vi "Get Instruments.vi"(8 "error in (no error)":errorcluster, 11 "Test Class in":refnum<class "Test Class.lvclass">) -> (0 "error out":errorcluster, 3 "Instruments":refnum<class "Instrument.lvclass">[](array[class]))   [LabVIEW 2017, in "Test Class.lvclass"]
uses:
  Test Class.lvclass
  Classes/Instruments/Instrument/Class/Instrument.lvclass
  Classes/Application/Class/Application.lvclass
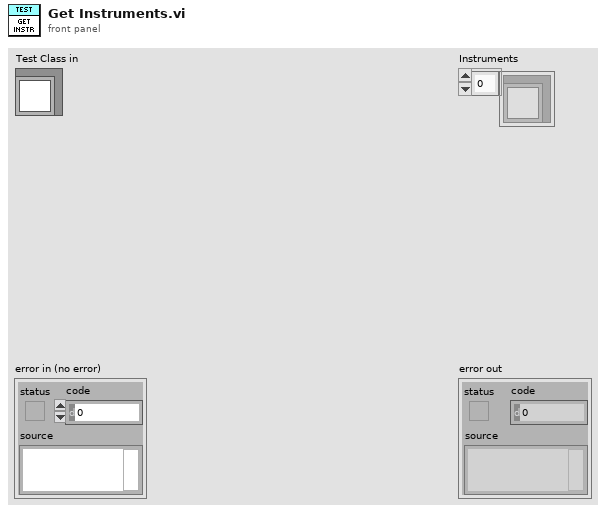
[diagram p1: front panel]
types:
  T1 = typedef "Application.lvlib/App Properties.lvclass/Class Properties -- Cluster.ctl" = cluster{"UUT Info":T2[], "Test Information":refnum<vi>, "Gold Board":refnum<class "Golden Board.lvclass">, "Test Recipe":refnum<class "Test Recipe.lvclass">, "Instruments":refnum<class "Instrument.lvclass">[], "Mode":T3, "Test Results":T4[], "Station Config":refnum<class "Station Config.lvclass">, "Variable Engine":refnum<class "Variable Engine.lvclass">}
  T2 = typedef "Application.lvlib/App Properties.lvclass/UUT Reference -- Cluster.ctl" = cluster{"Serial Number Reference":refnum<vi>, "Status Message Reference":refnum<vi>}
  T3 = typedef "Application.lvlib/Application.lvclass/Op Mode -- Enum.ctl" = u16
  T4 = typedef "Application.lvlib/App Properties.lvclass/Test Result -- Cluster.ctl" = cluster{"Position":i32, "Pass":bool, "Fail Codes":string}
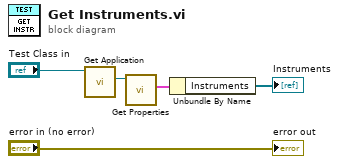
[diagram p0: block diagram]
diagram:
  n1 = call "Get Application.vi"("Test Class in"="Test Class in") -> ("Application.lvlib:Application.lvclass"=w2:refnum<class "Application.lvclass">)  [unwired: 9 in, 1 out]
  n2 = call "Get Properties.vi"("Acrobat Template in"=w2) -> ("Class Properties"=w4:T1)  [unwired: 8 in, 2 out]
  n3 = Unbundle By Name(w4) -> ("Instruments"=→"Instruments":refnum<class "Instrument.lvclass">[])
  "error out" <- "error in (no error)"
